vi "Read NombrePruebas 2.vi"(8 "error in (no error)":errorcluster, 11 "Equipo in":refnum<class "Equipo.lvclass">) -> (0 "error out":errorcluster, 2 "NombrePruebas":string[](array[string]), 3 "Equipo out":refnum<class "Equipo.lvclass">)   [LabVIEW 2019, in "Equipo.lvclass"]
uses:
  Equipo.lvclass
  Equipo.lvclass/Equipo.ctl
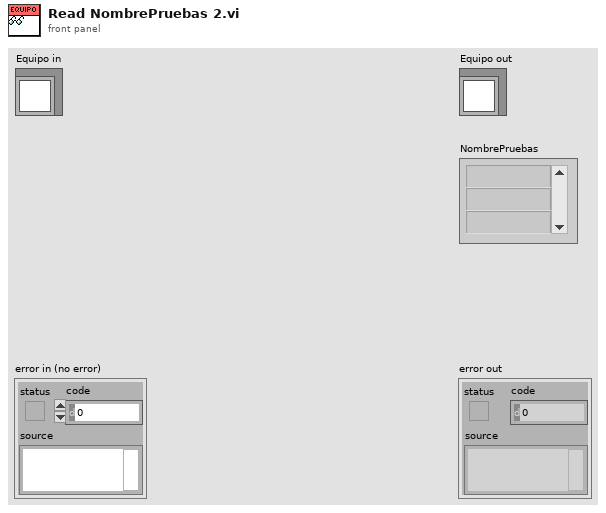
[diagram p1: front panel]
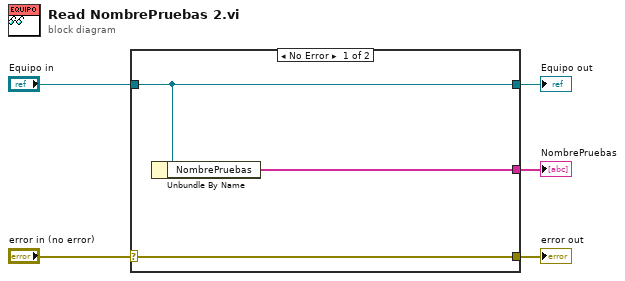
[diagram p0: block diagram]
diagram:
  n1 = case shown="No Error" "error in (no error)" {
    selector: "error in (no error)" -> [w8 w9]
    tunnel: [w8 w9] -> w4
    tunnel: [w7 w10] -> w2
    tunnel: "Equipo in" -> [w7 w10]
    tunnel: [w6 _] -> w1
    frame No Error {
      n2 = Unbundle By Name(w7) -> ("NombrePruebas"=w6:string[])
    }
    frame Error {
    }
  }
  "error out" <- w4
  "Equipo out" <- w2
  "NombrePruebas" <- w1
